vi "GUI.vi"(9 "Target Time (seconds)":dbl, 11 "Timer DVR":refnum<data-value>) -> ()   [LabVIEW 2018, in "Timer.lvclass"]
uses:
  Timer.lvclass
  Set Elapsed Time (seconds).vi
panel:
  out "Time Stamp":timestamp format="%^<%H:%M:%S>T"
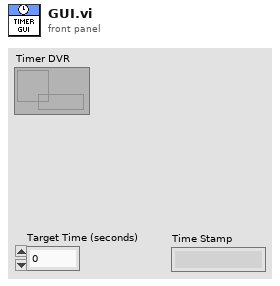
[diagram p1: front panel]
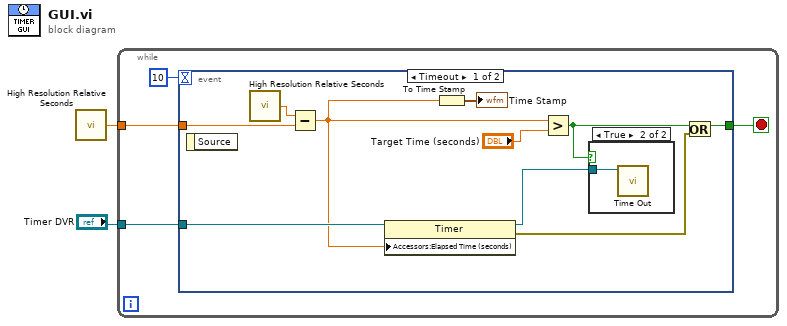
[diagram p0: block diagram]
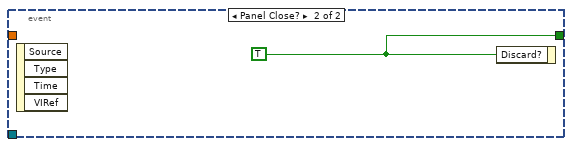
[diagram p3: hidden frame]
diagram:
  n1 = call <vilib>:"High Resolution Relative Seconds.vi"() -> ("relative seconds"=w2:dbl)
  n2 = while {
    tunnel: w2 -> [w5]
    tunnel: "Timer DVR" -> [w4]
    stop <- w3 stop-if-true
    n3 = event shown="[0] Timeout" {
      selector: _ -> [_ _]
      dyn-events: _ -> [_ _]
      timeout: 10 -> [_ _]
      tunnel: w5 -> [w15 _]
      tunnel: [w9 w18] -> w3
      tunnel: w4 -> [w12 _]
      event Timeout {
        n4 = event-data() -> ()  [unwired: 1 in, 1 out]
        n5 = call <vilib>:"High Resolution Relative Seconds.vi"() -> ("relative seconds"=w16:dbl)
        n6 = Subtract(x=w16, y=w15) -> (x-y=w11:dbl)
        n7 = property class="Timer"(reference=w12, "Accessors:Elapsed Time (seconds)"=w11) -> (reference out=w7:refnum<data-value>, error out=w8:errorcluster)  [unwired: 1 in]
        n8 = To Time Stamp(1:w11) -> (0:→"Time Stamp":timestamp)
        n9 = Greater?(x=w11, y="Target Time (seconds)") -> (0:w10:bool)
        n10 = case shown="True" w10 {
          tunnel: w7 -> [_ w17]
          frame False {
          }
          frame True {
            n11 = call "Time Out.vi"("Timer DVR"=w17) -> ()  [unwired: 11 in]
          }
        }
        n12 = Or(x=w10, y=w8) -> (x .or. y?=w9:bool)
      }
      event Panel Close? {
        w18 = TRUE ("Discard?")
        n13 = event-data() -> ()  [unwired: 1 in, 4 out]
        n14 = event-data("Discard?"=w18) -> ()  [unwired: 1 in, 1 out]
      }
    }
  }
